vi "Read.vi"   [LabVIEW 2024, in "Keithley 24XX.lvlib"]
doc: "Allows users to read one or more measurements from the DMM."
uses:
  <instrlib>/Keithley 24XX/Keithley 24XX.lvlib
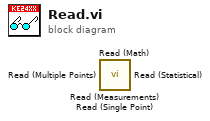
[diagram p0: block diagram]
diagram:
  n1 = call <instrlib>:"Read (Measurements).vi"() -> ()  [unwired: 9 in, 7 out]
  n2 = call <instrlib>:"Read (Math).vi"() -> ()  [unwired: 13 in, 3 out]
  n3 = call <instrlib>:"Read (Multiple Points).vi"() -> ()  [unwired: 9 in, 7 out]
  n4 = call <instrlib>:"Read (Statistical).vi"() -> ()  [unwired: 13 in, 3 out]
  n5 = call <instrlib>:"Read (Single Point).vi"() -> ()  [unwired: 9 in, 7 out]
